vi "PLC_EIP.vi"   [LabVIEW 2020]
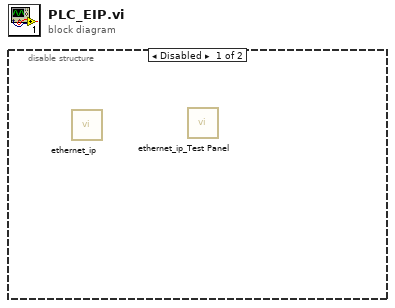
[diagram p0: block diagram]
diagram:
  n1 = disable-structure shown="Disabled" {
    frame Disabled {
      n2 = call "ethernet_ip.vi"() -> ()  [unwired: 7 in, 9 out]
      n3 = call "ethernet_ip_Test Panel.vi"() -> ()  [unwired: 11 in, 1 out]
    }
    frame Enabled {
    }
  }
